vi "analog read.vi"(8 "error in":errorcluster) -> (0 "error out":errorcluster, 2 "data":dbl[](array[numeric]))   [LabVIEW 2017]
uses:
  <vilib>/DAQmx/read.llb/DAQmx Read (Analog 1D Wfm NChan NSamp).vi
  <vilib>/Analysis/baseanly.llb/Mean (DBL).vi
  <vilib>/DAQmx/miscellaneous.llb/DAQmx Fill In Error Info.vi
  <vilib>/Analysis/NI_AALBase.lvlib
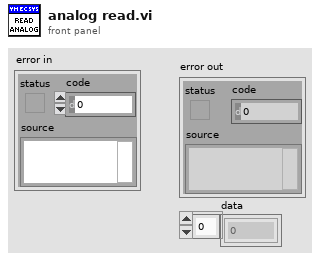
[diagram p1: front panel]
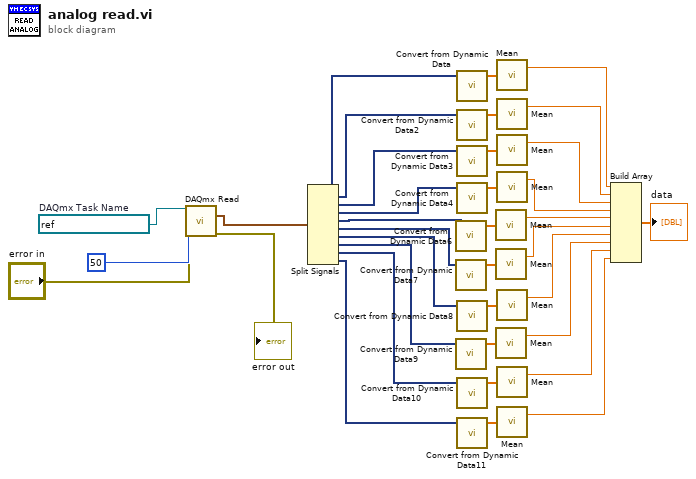
[diagram p0: block diagram]
diagram:
  w35 = refnum<k21> "Analog channel"  # DAQmx Task Name
  n1 = call-poly <vilib>:"DAQmx Read.vi"("task/channels in"=w35, "number of samples per channel"=50, "error in"="error in") -> ("data"=w34:waveform(dbl)[], "error out"=→"error out":errorcluster)  [unwired: 10 in, 1 out]
  n2 = Split Signals(w34) -> (w30:dynamicdata, w20:dynamicdata, w19:dynamicdata, w18:dynamicdata, w17:dynamicdata, w16:dynamicdata, w15:dynamicdata, w14:dynamicdata, w13:dynamicdata, w12:dynamicdata)  [unwired: 10 in]
  n3 = call "Convert from Dynamic Data6"("Dynamic Data Type"=w17) -> ("Array"=w26:dbl[])  [unwired: 3 in]
  n4 = call "Convert from Dynamic Data7"("Dynamic Data Type"=w16) -> ("Array"=w25:dbl[])  [unwired: 3 in]
  n5 = call "Convert from Dynamic Data9"("Dynamic Data Type"=w14) -> ("Array"=w23:dbl[])  [unwired: 3 in]
  n6 = call "Convert from Dynamic Data"("Dynamic Data Type"=w30) -> ("Array"=w31:dbl[])  [unwired: 3 in]
  n7 = call "Convert from Dynamic Data2"("Dynamic Data Type"=w20) -> ("Array"=w29:dbl[])  [unwired: 3 in]
  n8 = call "Convert from Dynamic Data3"("Dynamic Data Type"=w19) -> ("Array"=w28:dbl[])  [unwired: 3 in]
  n9 = call "Convert from Dynamic Data4"("Dynamic Data Type"=w18) -> ("Array"=w27:dbl[])  [unwired: 3 in]
  n10 = call "Convert from Dynamic Data8"("Dynamic Data Type"=w15) -> ("Array"=w24:dbl[])  [unwired: 3 in]
  n11 = call "Convert from Dynamic Data10"("Dynamic Data Type"=w13) -> ("Array"=w22:dbl[])  [unwired: 3 in]
  n12 = call "Convert from Dynamic Data11"("Dynamic Data Type"=w12) -> ("Array"=w21:dbl[])  [unwired: 3 in]
  n13 = call-poly <vilib>:"Mean.vi"("X"=w26) -> ("mean"=w7:dbl)  [unwired: 1 out]
  n14 = call-poly <vilib>:"Mean.vi"("X"=w25) -> ("mean"=w6:dbl)  [unwired: 1 out]
  n15 = call-poly <vilib>:"Mean.vi"("X"=w23) -> ("mean"=w4:dbl)  [unwired: 1 out]
  n16 = call-poly <vilib>:"Mean.vi"("X"=w31) -> ("mean"=w11:dbl)  [unwired: 1 out]
  n17 = call-poly <vilib>:"Mean.vi"("X"=w29) -> ("mean"=w10:dbl)  [unwired: 1 out]
  n18 = call-poly <vilib>:"Mean.vi"("X"=w28) -> ("mean"=w9:dbl)  [unwired: 1 out]
  n19 = call-poly <vilib>:"Mean.vi"("X"=w27) -> ("mean"=w8:dbl)  [unwired: 1 out]
  n20 = call-poly <vilib>:"Mean.vi"("X"=w24) -> ("mean"=w5:dbl)  [unwired: 1 out]
  n21 = call-poly <vilib>:"Mean.vi"("X"=w22) -> ("mean"=w3:dbl)  [unwired: 1 out]
  n22 = call-poly <vilib>:"Mean.vi"("X"=w21) -> ("mean"=w2:dbl)  [unwired: 1 out]
  n23 = Build Array(w11, w10, w9, w8, w7, w6, w5, w4, w3, w2) -> (→"data":dbl[])
